vi "window parameters.vi"(0 "window":T1(ring)) -> (1 "ENBW":dbl format="%0.2f", 2 "Coherent Gain":dbl format="%0.2f", 3 "6dB BW":dbl format="%0.2f")   [LabVIEW 2017, in "NI_AALPro.lvlib"]
uses:
  NI_AALPro.lvlib
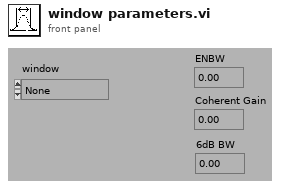
[diagram p1: front panel]
types:
  T1 = enum16{"None ", "Hanning", "Hamming", "Blackman-Harris", "Exact Blackman", "Blackman", "Flat Top", "4 Term B-Harris ", "7 Term B-Harris", "Low Sidelobe"}
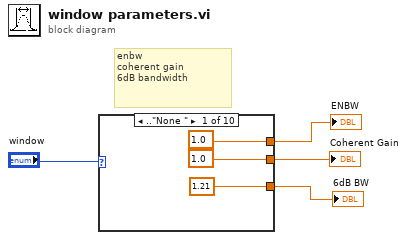
[diagram p0: block diagram]
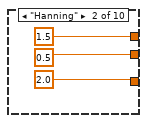
[diagram p2: hidden frame]
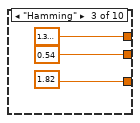
[diagram p3: hidden frame]
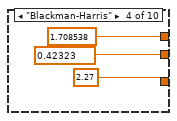
[diagram p4: hidden frame]
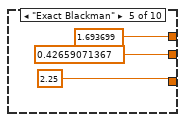
[diagram p5: hidden frame]
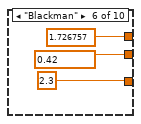
[diagram p6: hidden frame]
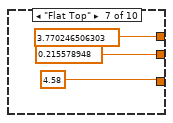
[diagram p7: hidden frame]
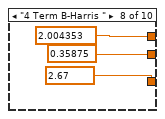
[diagram p8: hidden frame]
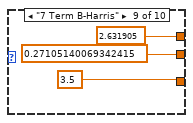
[diagram p9: hidden frame]
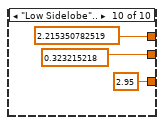
[diagram p10: hidden frame]
diagram:
  # "enbw\ncoherent gain\n6dB bandwidth"
  n1 = case shown="..\"None \"" "window" {
    tunnel: [1.0 0.5 0.54 0.42323 0.42659071367 0.42 0.215578948 0.35875 0.27105140069342415 0.323215218] -> w3
    tunnel: [1.0 1.5 1.362826 1.708538 1.693699 1.726757 3.770246506303 2.004353 2.631905 2.215350782519] -> w4
    tunnel: [1.21 2.0 1.82 2.27 2.25 2.3 4.58 2.67 3.5 2.95] -> w2
    frame .."None " {
    }
    frame "Hanning" {
    }
    frame "Hamming" {
    }
    frame "Blackman-Harris" {
    }
    frame "Exact Blackman" {
    }
    frame "Blackman" {
    }
    frame "Flat Top" {
    }
    frame "4 Term B-Harris " {
    }
    frame "7 Term B-Harris" {
    }
    frame "Low Sidelobe".. {
    }
  }
  "ENBW" <- w4
  "Coherent Gain" <- w3
  "6dB BW" <- w2
